vi "Wait for Message.vi"(8 "error in":errorcluster, 10 "Timeout":i32 format="%d ms", 11 "Win32 Event in":refnum<class "Win32 Event.lvclass">) -> (0 "error out":errorcluster, 2 "Timed Out":bool, 3 "Win32 Event out":refnum<class "Win32 Event.lvclass">)   [LabVIEW 2020, in "PCANBasic.lvlib" / "Win32 Event.lvclass"]
uses:
  Win32 Event.lvclass
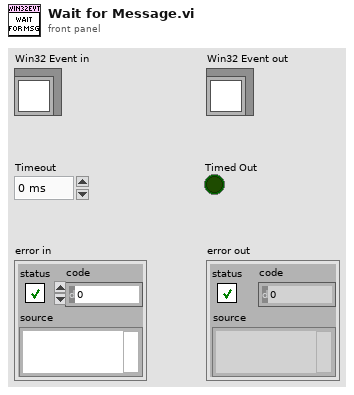
[diagram p1: front panel]
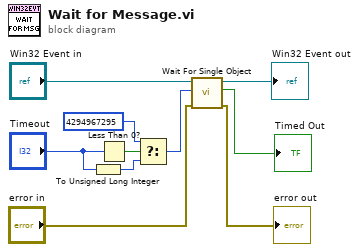
[diagram p0: block diagram]
diagram:
  n1 = To Unsigned Long Integer(number="Timeout") -> (unsigned 32bit integer=w2:u32)
  n2 = Less Than 0?(x="Timeout") -> (x < 0?=w5:bool)
  n3 = Select(t=u32 4294967295 ("Timeout"), s=w5, f=w2) -> (s? t:f=w1:u32)
  n4 = call "Wait For Single Object.vi"("error in"="error in", "Timeout"=w1, "Win32 Event in"="Win32 Event in") -> ("error out"=→"error out":errorcluster, "Timed Out"=→"Timed Out":bool, "Win32 Event out"=→"Win32 Event out":refnum<class "Win32 Event.lvclass">)  [unwired: 6 in]
